vi "Excel_Insert_Footer.vi"(0 "Excel._Worksheet":refnum<k7>, 1 "font":T1 {"font size" format="%0.2f"}, 5 "left footer text":string, 7 "center footer text":string, 9 "right footer text":string, 11 "error in (no error)":errorcluster) -> (15 "error out":errorcluster)   [LabVIEW 2020, in "NI_ReportGenerationToolkit.lvlib"]
uses:
  <vilib>/addons/_office/NI_ReportGenerationToolkit.lvlib
  <vilib>/Utility/NIReport.llb/NI_ReportGenerationCore.lvlib
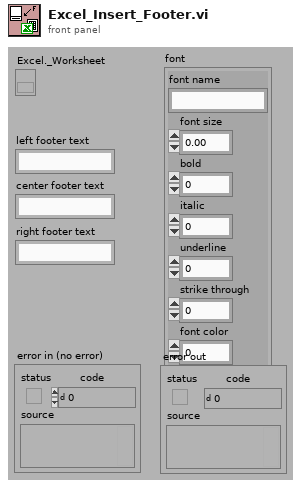
[diagram p1: front panel]
types:
  T1 = cluster{"font name":string, "font size":dbl, "bold":u16, "italic":u16, "underline":u16, "strike through":u16, "font color":i32}
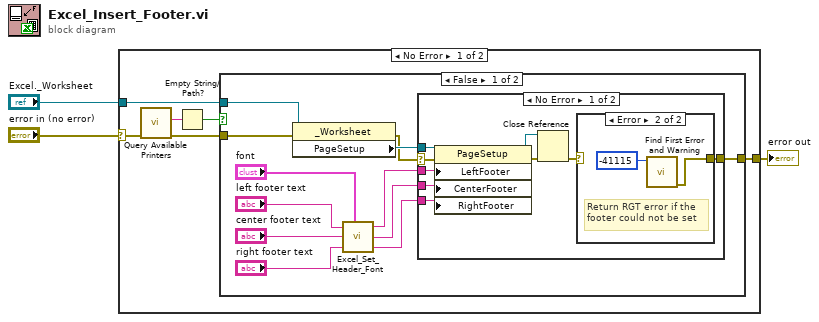
[diagram p0: block diagram]
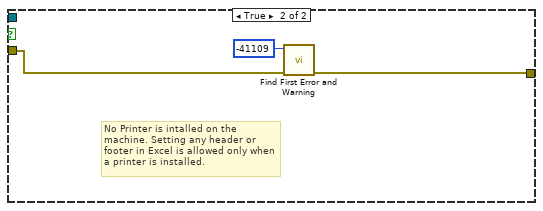
[diagram p4: hidden frame]
diagram:
  n1 = case shown="No Error" "error in (no error)" {
    selector: "error in (no error)" -> [w4 w38]
    tunnel: [w9 w38] -> w3
    tunnel: "Excel._Worksheet" -> [w8 _]
    frame No Error {
      n2 = call <vilib>:"Query Available Printers.vi"("error in (no error)"=w4) -> ("error out"=w7:errorcluster, "default printer"=w6:string)  [unwired: 9 out]
      n3 = Empty String/Path?(string/path=w6) -> (empty?=w5:bool)
      n4 = case shown="False" w5 {
        tunnel: [w14 w36] -> w9
        tunnel: w8 -> [w12 _]
        tunnel: w7 -> [w11 w35]
        frame False {
          n5 = property class="_Worksheet"(reference=w12, error in=w11) -> (error out=w10:errorcluster, "PageSetup"=w13:refnum<k7>)  [unwired: 1 out]
          n6 = call <vilib>:"Excel_Set_Header_Font.vi"("left footer text in"="left footer text", "font"="font", "center footer text in"="center footer text", "right footer text in"="right footer text") -> ("left footer text out"=w19:string, "center footer text out"=w20:string, "right footer text out"=w21:string)  [unwired: 3 out]
          n7 = case shown="No Error" w10 {
            selector: w10 -> [w24 w34]
            tunnel: w21 -> [w30 _]
            tunnel: w20 -> [w29 _]
            tunnel: w19 -> [w28 _]
            tunnel: [w22 w34] -> w14
            tunnel: w13 -> [w25 _]
            frame No Error {
              n8 = property class="PageSetup"(reference=w25, error in=w24, "LeftFooter"=w28, "CenterFooter"=w29, "RightFooter"=w30) -> (reference out=w27:refnum<k7>, error out=w26:errorcluster)
              n9 = Close Reference(reference=w27, error in (no error)=w26) -> (error out=w23:errorcluster)
              n10 = case shown="Error" w23 {
                selector: w23 -> [w31 _]
                tunnel: [w31 w33] -> w22
                frame No Error {
                }
                frame Error {
                  # "Return RGT error if the\nfooter could not be set"
                  n11 = call <vilib>:"Find First Error and Warning.vi"("error code"=-41115) -> ("error out"=w33:errorcluster)  [unwired: 1 in, 5 out]
                }
              }
            }
            frame Error {
            }
          }
        }
        frame True {
          # "No Printer is intalled on the machine. Setting any header or footer in Excel is allowed only when a printer is installed."
          n12 = call <vilib>:"Find First Error and Warning.vi"("error in (no error)"=w35, "error code"=-41109) -> ("error out"=w36:errorcluster)  [unwired: 5 out]
        }
      }
    }
    frame Error {
    }
  }
  "error out" <- w3
